vi "Teleop.vi"(0 "Call Context":T10) -> (6 "SubState 3":T4, 8 "SubState 4":T4, 9 "SubState 5":T9, 11 "Loop 3 Data":T5, 13 "Loop 4 Data":T3, 14 "SubState 0":T4=enum."driver control", 15 "Loop 1 Data":T7, 16 "Loop 0 Data":T8, 17 "SubState 1":T4, 18 "Loop 2 Data":T6, 19 "SubState 2":T4)   [LabVIEW 2013]
uses:
  typedefs/subStates.ctl
  <vilib>/Rock Robotics/WPI/DriverStation/WPI_DriverStationDerivedRobotMode.ctl
  typedefs/singleUseSubstate.ctl
  typedefs/Loop Datatypes/Loop 0 Datatype.ctl
  typedefs/Loop Datatypes/Loop 1 Datatype.ctl
  typedefs/Loop Datatypes/Loop 2 Datatype.ctl
  typedefs/Loop Datatypes/Loop 3 Datatype.ctl
  typedefs/Loop Datatypes/Loop 4 Datatype.ctl
  <vilib>/Rock Robotics/WPI/Joystick/WPI_JoystickDevRef.ctl
  <vilib>/Rock Robotics/WPI/Joystick/WPI_JoystickDeviceEnum.ctl
  typedefs/fg_typedef.ctl
  typedefs/vision enable.ctl
  <vilib>/Rock Robotics/WPI/Joystick/WPI_JoystickGetSetRefNum.vi
panel:
  out "JS3":T1
  out "Drive to DC":bool
  out "JS1":T1
  out "JS2":T1
  out "Exit Value":i32=-1
  # "Loop Data and Substates"
  # "Drive Loop"
  # "Shooter Pneumatics Loop"
  # "Pickup/Passing Belts Loop"
  # "Pickup Arm Loop"
  # "Shifter Loop"
  # "Latch Loop"
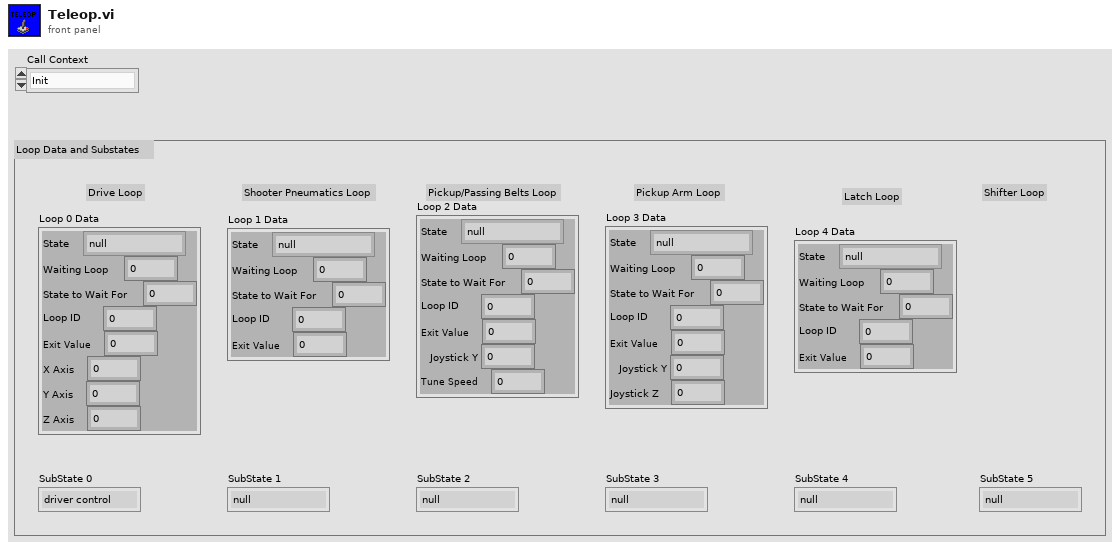
[diagram p1: front panel]
types:
  T1 = typedef "WPI_JoystickDevRef.ctl" = cluster{"Device":T2}
  T2 = typedef "WPI_JoystickDeviceEnum.ctl" = enum16{"USB 1", "USB 2", "USB 3", "USB 4", "Kinect 1", "Kinect 2"}
  T3 = typedef "Loop 4 Datatype.ctl" = cluster{"State":T4, "Waiting Loop":i32, "State to Wait For":i32, "Loop ID":i32, "Exit Value":i32}
  T4 = typedef "subStates.ctl" = enum16{"null", "wait", "driver control", "auto", "manual override", "hold position", "rotate", "pickup", "pass", "load", "goto shoot", "shoot", "end"}
  T5 = typedef "Loop 3 Datatype.ctl" = cluster{"State":T4, "Waiting Loop":i32, "State to Wait For":i32, "Loop ID":i32, "Exit Value":i32, "Joystick Y":dbl, "Joystick Z":dbl}
  T6 = typedef "Loop 2 Datatype.ctl" = cluster{"State":T4, "Waiting Loop":i32, "State to Wait For":i32, "Loop ID":i32, "Exit Value":i32, "Joystick Y":dbl, "Tune Speed":dbl}
  T7 = typedef "Loop 1 Datatype.ctl" = cluster{"State":T4, "Waiting Loop":i32, "State to Wait For":i32, "Loop ID":i32, "Exit Value":i32}
  T8 = typedef "Loop 0 Datatype.ctl" = cluster{"State":T4, "Waiting Loop":i32, "State to Wait For":i32, "Loop ID":i32, "Exit Value":i32, "X Axis":dbl, "Y Axis":dbl, "Z Axis":dbl}
  T9 = typedef "singleUseSubstate.ctl" = enum16{"null", "wait", "shift high", "shift low"}
  T10 = typedef "WPI_DriverStationDerivedRobotMode.ctl" = enum16{"Init", "Execute", "Stop"}
  T11 = cluster{"axis 1 (x)":dbl, "axis 2 (y)":dbl, "axis 3 (throttle)":dbl, "axis 4":dbl, "axis 5":dbl, "axis 6":dbl}
  T12 = typedef "WPI_EncoderDevRef.ctl" = cluster{"DevStatus":errorcluster, "EncoderIndex":T13, "CounterIndex":T14, "DistancePerCount":dbl, "Decoding Type":T15}
  T13 = typedef "FPGA_EncoderIdx.ctl" = enum8{"Enc 0", "Enc 1", "Enc 2", "Enc 3", "Invalid"}
  T14 = typedef "FPGA_CounterCtrSystemIndex.ctl" = enum8{"Ctr 0", "Ctr 1", "Ctr 2", "Ctr 3", "Ctr 4", "Ctr 5", "Ctr 6", "Ctr 7", "Invalid"}
  T15 = typedef "WPI_EncoderType.ctl" = enum16{"1x", "2x", "4x"}
  T16 = typedef "vision enable.ctl" = enum16{"Enable", "Disable", "Stop"}
  T17 = typedef "fg_typedef.ctl" = enum16{"Get", "Set"}
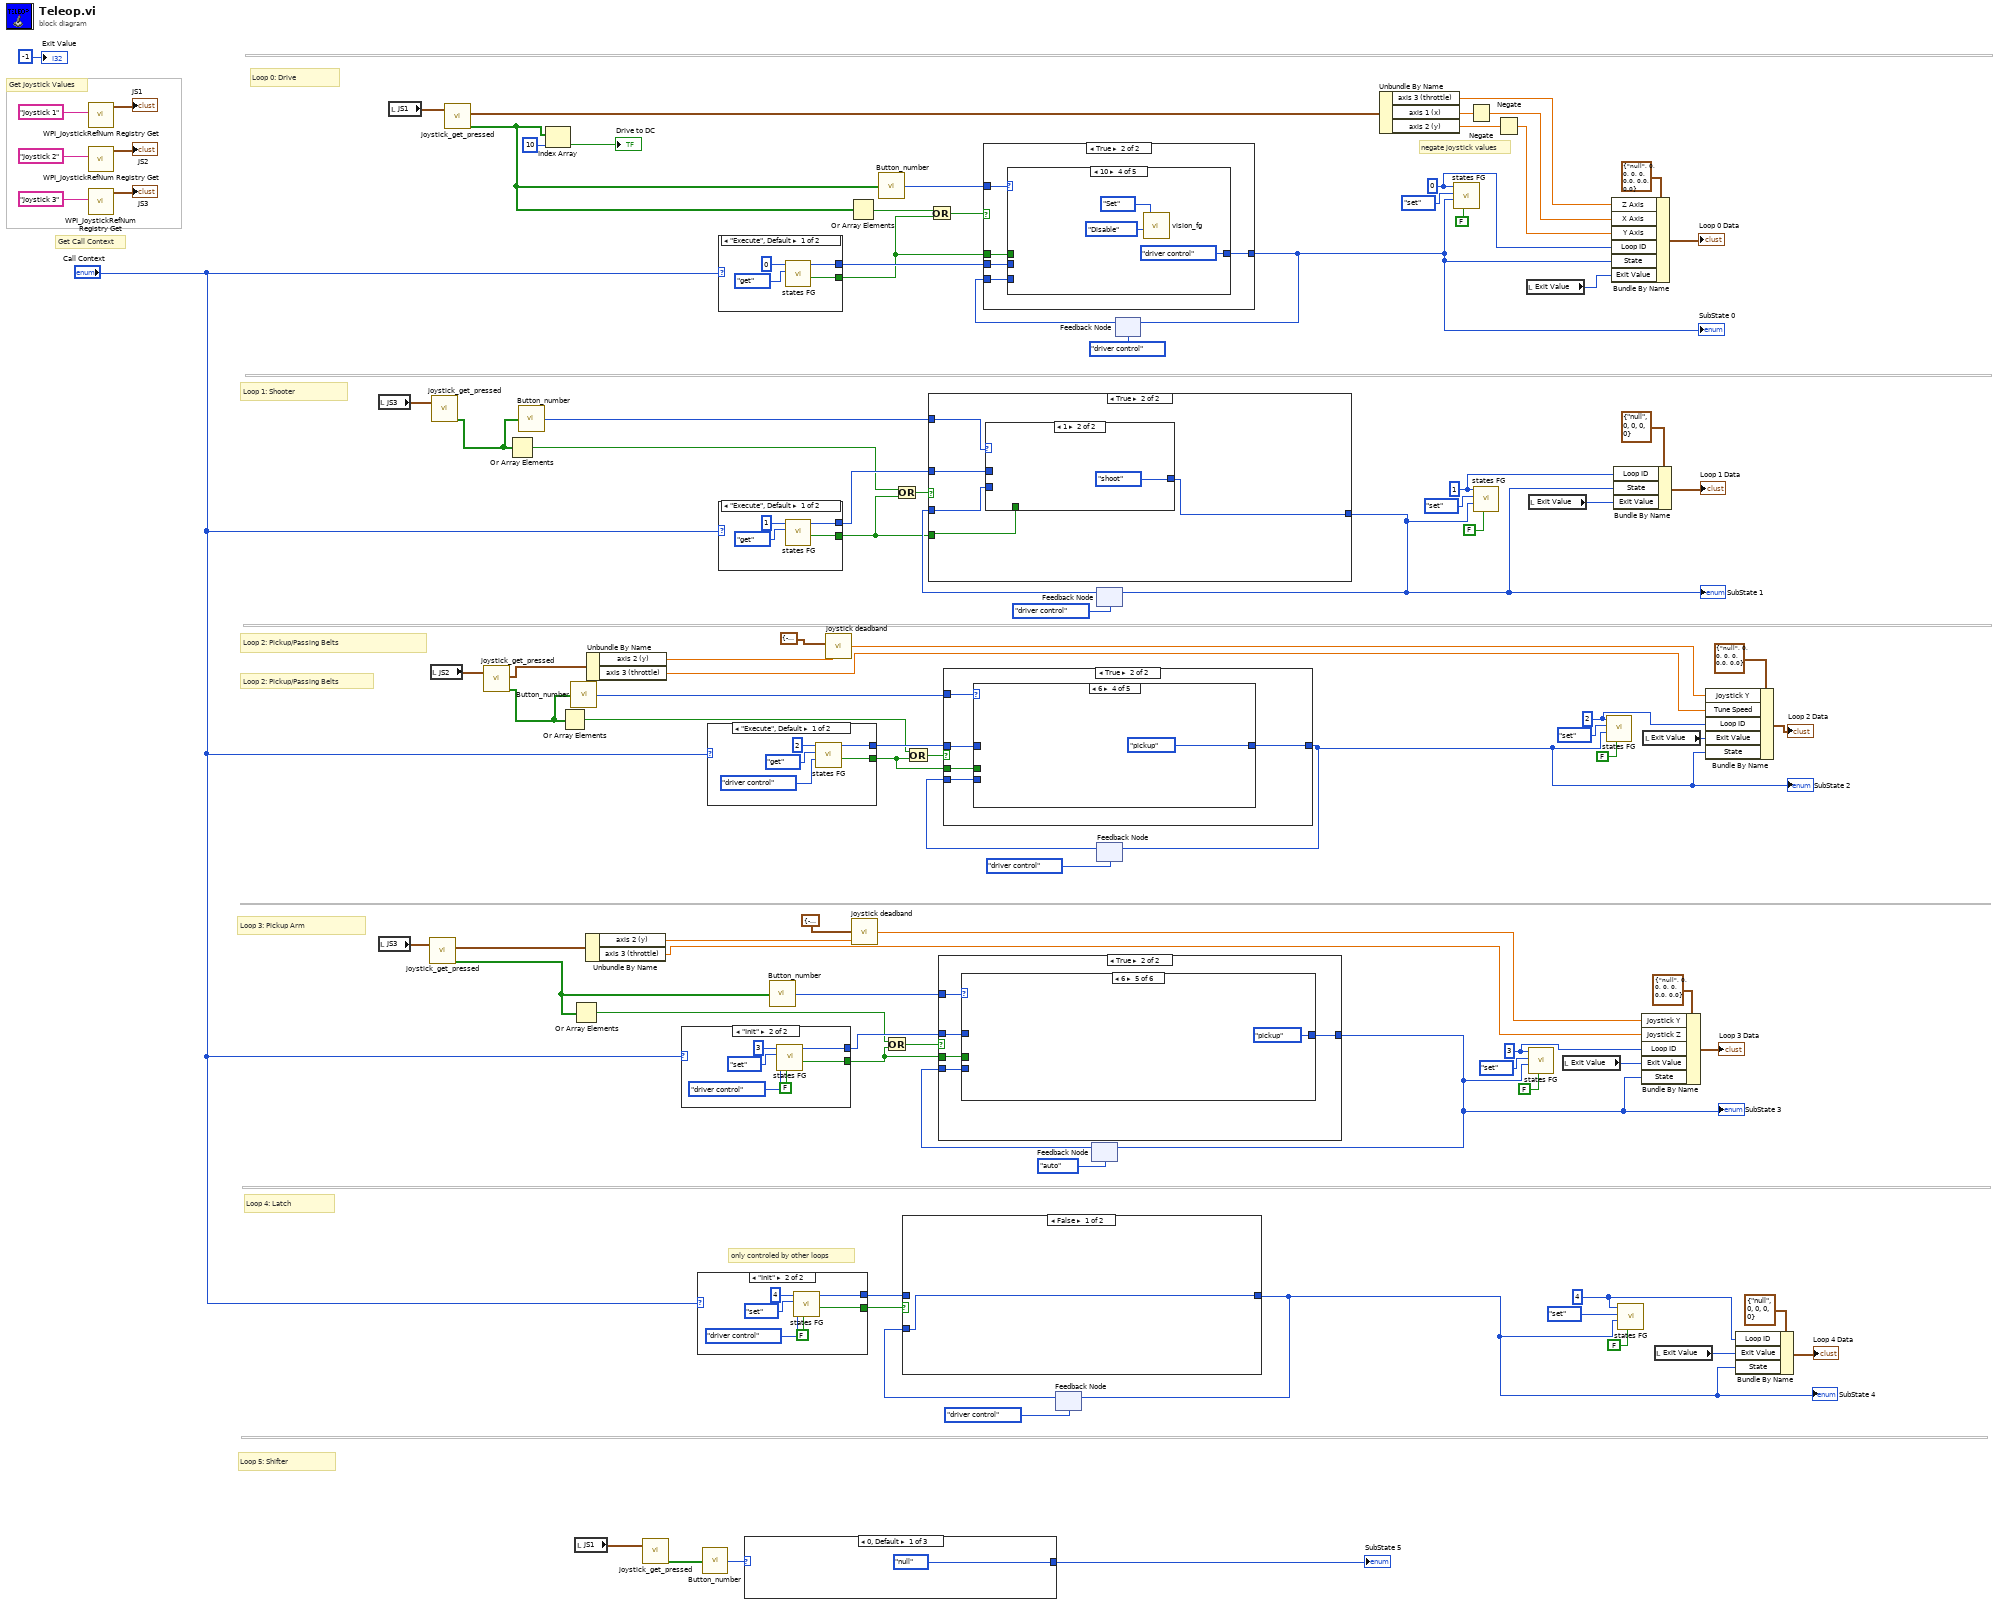
[diagram p0: block diagram]
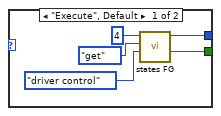
[diagram p3: hidden frame]
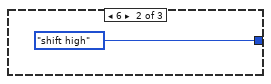
[diagram p4: hidden frame]
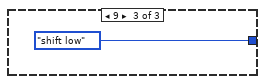
[diagram p5: hidden frame]
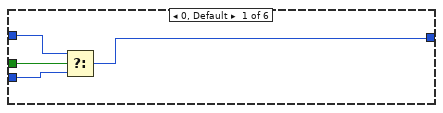
[diagram p7: hidden frame]
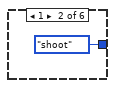
[diagram p8: hidden frame]
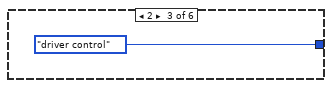
[diagram p9: hidden frame]
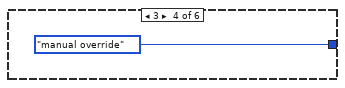
[diagram p10: hidden frame]
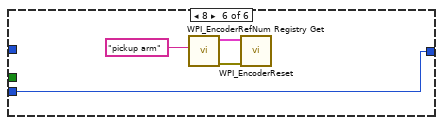
[diagram p11: hidden frame]
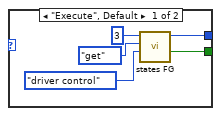
[diagram p12: hidden frame]
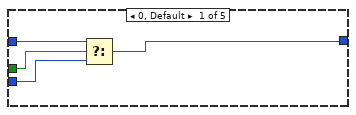
[diagram p14: hidden frame]
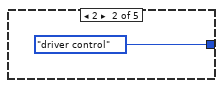
[diagram p15: hidden frame]
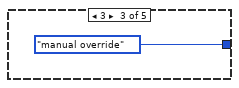
[diagram p16: hidden frame]
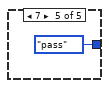
[diagram p17: hidden frame]
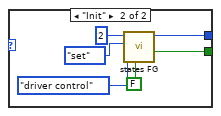
[diagram p18: hidden frame]
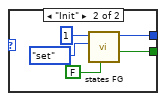
[diagram p19: hidden frame]
diagram:
  w9 = 4 ("Loop ID")
  w77 = 3 ("Loop ID")
  w78 = 2 ("Loop ID")
  w87 = 1 ("Loop ID")
  w89 = 0 ("Loop ID")
  # "only controled by other loops"
  # "Loop 2: Pickup/Passing Belts"
  # "negate joystick values"
  # "Get Call Context"
  # "Get Joystick Values"
  # "Loop 4: Latch"
  # "Loop 3: Pickup Arm"
  # "Loop 5: Shifter"
  # "Loop 2: Pickup/Passing Belts"
  # "Loop 1: Shooter"
  # "Loop 0: Drive"
  n1 = call <vilib>:"WPI_JoystickRefNum Registry Get.vi"("refnum name"="Joystick 1") -> ("JoystickDevRef"=→"JS1":T1)  [unwired: 9 in, 1 out]
  n2 = call <vilib>:"WPI_JoystickRefNum Registry Get.vi"("refnum name"="Joystick 2") -> ("JoystickDevRef"=→"JS2":T1)  [unwired: 9 in, 1 out]
  n3 = call <vilib>:"WPI_JoystickRefNum Registry Get.vi"("refnum name"="Joystick 3") -> ("JoystickDevRef"=→"JS3":T1)  [unwired: 9 in, 1 out]
  n4 = local read "JS3"() -> (w53:T1)
  n5 = local read "JS3"() -> (w38:T1)
  n6 = local read "JS1"() -> (w54:T1)
  n7 = call "joystick_get_pressed.vi"("JoystickDevRef 2"=w38) -> ("Axes"=w42:T11, "Buttons Pressed?"=w18:bool[])  [unwired: 1 in, 2 out]
  n8 = local read "JS2"() -> (w25:T1)
  n9 = call "joystick_get_pressed.vi"("JoystickDevRef 2"=w53) -> ("Buttons Pressed?"=w20:bool[])  [unwired: 1 in, 3 out]
  n10 = call "joystick_get_pressed.vi"("JoystickDevRef 2"=w54) -> ("Axes"=w58:T11, "Buttons Pressed?"=w33:bool[])  [unwired: 1 in, 2 out]
  n11 = call "joystick_get_pressed.vi"("JoystickDevRef 2"=w25) -> ("Axes"=w5:T11, "Buttons Pressed?"=w6:bool[])  [unwired: 1 in, 2 out]
  n12 = Or Array Elements(Boolean array=w20) -> (logical OR=w45:bool)
  n13 = call "Button_number.vi"("Button Array"=w20) -> ("Button Pressed"=w47:i32)
  n14 = Index Array(array=w33, index=10) -> (element=→"Drive to DC":bool)
  n15 = Or Array Elements(Boolean array=w6) -> (logical OR=w24:bool)
  n16 = call "Button_number.vi"("Button Array"=w6) -> ("Button Pressed"=w23:i32)
  n17 = Or Array Elements(Boolean array=w18) -> (logical OR=w41:bool)
  n18 = local read "JS1"() -> (w28:T1)
  n19 = Unbundle By Name(w42) -> ("axis 2 (y)"=w36:dbl, "axis 3 (throttle)"=w1:dbl)
  n20 = Unbundle By Name(w5) -> ("axis 2 (y)"=w17:dbl, "axis 3 (throttle)"=w3:dbl)
  n21 = call "joystick_get_pressed.vi"("JoystickDevRef 2"=w28) -> ("Buttons Pressed?"=w30:bool[])  [unwired: 1 in, 3 out]
  n22 = case shown="\"Init\"" "Call Context" {
    tunnel: [w108 w114] -> w39
    tunnel: [w106 w111] -> w75
    frame "Execute", Default {
      n23 = call "states FG.vi"("subState in"=subStates."driver control", "menu (get)"=enum16{"set", "get"}."get", "Loop ID"=3) -> ("exit out"=w108:bool, "subState out"=w106:T4)  [unwired: 5 in, 2 out]
    }
    frame "Init" {
      n24 = call "states FG.vi"("exit in"=FALSE, "subState in"=subStates."driver control", "menu (get)"=enum16{"set", "get"}."set", "Loop ID"=3) -> ("exit out"=w114:bool, "subState out"=w111:T4)  [unwired: 4 in, 2 out]
    }
  }
  n25 = case shown="\"Init\"" "Call Context" {
    tunnel: [w119 w125] -> w7
    tunnel: [w117 w122] -> w11
    frame "Execute", Default {
      n26 = call "states FG.vi"("subState in"=subStates."driver control", "menu (get)"=enum16{"set", "get"}."get", "Loop ID"=4) -> ("exit out"=w119:bool, "subState out"=w117:T4)  [unwired: 5 in, 2 out]
    }
    frame "Init" {
      n27 = call "states FG.vi"("exit in"=FALSE, "subState in"=subStates."driver control", "menu (get)"=enum16{"set", "get"}."set", "Loop ID"=4) -> ("exit out"=w125:bool, "subState out"=w122:T4)  [unwired: 4 in, 2 out]
    }
  }
  n28 = call "Button_number.vi"("Button Array"=w30) -> ("Button Pressed"=w29:i32)
  n29 = case shown="\"Execute\", Default" "Call Context" {
    tunnel: [w130 w136] -> w44
    tunnel: [w128 w133] -> w94
    frame "Execute", Default {
      n30 = call "states FG.vi"("subState in"=subStates."driver control", "menu (get)"=enum16{"set", "get"}."get", "Loop ID"=2) -> ("exit out"=w130:bool, "subState out"=w128:T4)  [unwired: 5 in, 2 out]
    }
    frame "Init" {
      n31 = call "states FG.vi"("exit in"=FALSE, "subState in"=subStates."driver control", "menu (get)"=enum16{"set", "get"}."set", "Loop ID"=2) -> ("exit out"=w136:bool, "subState out"=w133:T4)  [unwired: 4 in, 2 out]
    }
  }
  n32 = case shown="\"Execute\", Default" "Call Context" {
    tunnel: [w140 w145] -> w51
    tunnel: [w139 w143] -> w92
    frame "Execute", Default {
      n33 = call "states FG.vi"("menu (get)"=enum16{"set", "get"}."get", "Loop ID"=0) -> ("exit out"=w140:bool, "subState out"=w139:T4)  [unwired: 6 in, 2 out]
    }
    frame "Init" {
      n34 = call "states FG.vi"("exit in"=FALSE, "menu (get)"=enum16{"set", "get"}."set", "Loop ID"=0) -> ("exit out"=w145:bool, "subState out"=w143:T4)  [unwired: 5 in, 2 out]
    }
  }
  n35 = case shown="\"Execute\", Default" "Call Context" {
    tunnel: [w149 w154] -> w48
    tunnel: [w148 w152] -> w91
    frame "Execute", Default {
      n36 = call "states FG.vi"("menu (get)"=enum16{"set", "get"}."get", "Loop ID"=1) -> ("exit out"=w149:bool, "subState out"=w148:T4)  [unwired: 6 in, 2 out]
    }
    frame "Init" {
      n37 = call "states FG.vi"("exit in"=FALSE, "menu (get)"=enum16{"set", "get"}."set", "Loop ID"=1) -> ("exit out"=w154:bool, "subState out"=w152:T4)  [unwired: 5 in, 2 out]
    }
  }
  n38 = case shown="0, Default" w29 {
    tunnel: [singleUseSubstate."null" ("Enum") singleUseSubstate."shift high" ("Enum") singleUseSubstate."shift low" ("Enum")] -> w67
    frame 0, Default {
    }
    frame 6 {
    }
    frame 9 {
    }
  }
  "SubState 5" <- w67
  n39 = call "Button_number.vi"("Button Array"=w18) -> ("Button Pressed"=w40:i32)
  n40 = call "joystick deadband.vi"("Joystick In"=w17, "Deadband Range"=cluster{"Deadband Min":dbl, "Deadband Max":dbl} {"Deadband Min"=-0.05, "Deadband Max"=0.05}) -> ("Joystick Out"=w4:dbl)  [unwired: 4 in]
  n41 = Or Array Elements(Boolean array=w33) -> (logical OR=w52:bool)
  n42 = call "joystick deadband.vi"("Joystick In"=w36, "Deadband Range"=cluster{"Deadband Min":dbl, "Deadband Max":dbl} {"Deadband Min"=-0.05, "Deadband Max"=0.05}) -> ("Joystick Out"=w2:dbl)  [unwired: 4 in]
  n43 = call "Button_number.vi"("Button Array"=w33) -> ("Button Pressed"=w57:i32)
  n44 = Or(x=w41, y=w39) -> (x .or. y?=w43:bool)
  n45 = Or(x=w45, y=w48) -> (x .or. y?=w49:bool)
  n46 = Or(x=w24, y=w44) -> (x .or. y?=w46:bool)
  n47 = Or(x=w52, y=w51) -> (x .or. y?=w50:bool)
  n48 = feedback #1(subStates."driver control" ("Drive SubState")) -> (w14:T4)
  n49 = case shown="False" w7 {
    tunnel: w14 -> [w160 _]
    tunnel: [w160 w161] -> w37
    tunnel: w11 -> [_ w161]
    frame False {
    }
    frame True {
    }
  }
  "SubState 4" <- w37
  n50 = feedback-in #1(w37) -> ()
  n51 = feedback #2(subStates."auto" ("Drive SubState")) -> (w72:T4)
  n52 = case shown="True" w43 {
    tunnel: w72 -> [w162 w163]
    tunnel: [w162 w164] -> w59
    tunnel: w75 -> [_ w165]
    tunnel: w40 -> [_ w167]
    tunnel: w39 -> [_ w166]
    frame False {
    }
    frame True {
      n53 = case shown="6" w167 {
        tunnel: w166 -> [w171 _ _ _ _ _]
        tunnel: w163 -> [w170 _ _ _ _ w179]
        tunnel: w165 -> [w169 _ _ _ _ _]
        tunnel: [w168 subStates."shoot" ("Drive SubState") subStates."driver control" ("Drive SubState") subStates."manual override" ("Drive SubState") subStates."pickup" ("Drive SubState") w179] -> w164
        frame 0, Default {
          n54 = Select(t=w169, s=w171, f=w170) -> (s? t:f=w168:T4)
        }
        frame 1 {
        }
        frame 2 {
        }
        frame 3 {
        }
        frame 6 {
        }
        frame 8 {
          n55 = call <vilib>:"WPI_EncoderRefNum Registry Get.vi"("refnum name"="pickup arm") -> ("error out"=w177:errorcluster, "EncoderDevRef"=w176:T12)  [unwired: 9 in]
          n56 = call <vilib>:"WPI_EncoderReset.vi"("error in (no error)"=w177, "EncoderDevRef"=w176) -> ()  [unwired: 8 in, 2 out]
        }
      }
    }
  }
  "SubState 3" <- w59
  n57 = feedback-in #2(w59) -> ()
  n58 = feedback #3(subStates."driver control" ("Drive SubState")) -> (w93:T4)
  n59 = case shown="True" w49 {
    tunnel: w93 -> [w180 w184]
    tunnel: [w180 w181] -> w60
    tunnel: w91 -> [_ w185]
    tunnel: w47 -> [_ w183]
    tunnel: w48 -> [_ w182]
    frame False {
      # "nothing pressed here, move along"
    }
    frame True {
      n60 = case shown="1" w183 {
        tunnel: w185 -> [w188 _]
        tunnel: w184 -> [w187 _]
        tunnel: [w186 subStates."shoot" ("Drive SubState")] -> w181
        tunnel: w182 -> [w189 _]
        frame 0, Default {
          n61 = Select(t=w188, s=w189, f=w187) -> (s? t:f=w186:T4)
        }
        frame 1 {
        }
      }
    }
  }
  "SubState 1" <- w60
  n62 = feedback-in #3(w60) -> ()
  n63 = feedback #4(subStates."driver control" ("Drive SubState")) -> (w97:T4)
  n64 = case shown="True" w46 {
    tunnel: w97 -> [w191 w193]
    tunnel: [w191 w192] -> w16
    tunnel: w94 -> [_ w194]
    tunnel: w23 -> [_ w196]
    tunnel: w44 -> [_ w195]
    frame False {
    }
    frame True {
      n65 = case shown="6" w196 {
        tunnel: w195 -> [w200 _ _ _ _]
        tunnel: w194 -> [w199 _ _ _ _]
        tunnel: w193 -> [w198 _ _ _ _]
        tunnel: [w197 subStates."driver control" ("Drive SubState") subStates."manual override" ("Drive SubState") subStates."pickup" ("Drive SubState") subStates."pass" ("Drive SubState")] -> w192
        frame 0, Default {
          n66 = Select(t=w199, s=w200, f=w198) -> (s? t:f=w197:T4)
        }
        frame 2 {
        }
        frame 3 {
        }
        frame 6 {
        }
        frame 7 {
        }
      }
    }
  }
  "SubState 2" <- w16
  n67 = feedback-in #4(w16) -> ()
  n68 = feedback #5(subStates."driver control" ("Drive SubState")) -> (w99:T4)
  n69 = case shown="True" w50 {
    tunnel: w99 -> [w205 w207]
    tunnel: [w205 w206] -> w27
    tunnel: w92 -> [_ w208]
    tunnel: w57 -> [_ w210]
    tunnel: w51 -> [_ w209]
    frame False {
      # "keep current state, no change necessary"
    }
    frame True {
      n70 = case shown="10" w210 {
        tunnel: w209 -> [w214 _ _ _ _]
        tunnel: w208 -> [w213 _ _ _ _]
        tunnel: w207 -> [w212 w219 _ _ _]
        tunnel: [w211 w215 subStates."goto shoot" ("Drive SubState") subStates."driver control" ("Drive SubState") subStates."driver control" ("Drive SubState")] -> w206
        frame 0, Default {
          n71 = Select(t=w213, s=w214, f=w212) -> (s? t:f=w211:T4)
        }
        frame 7 {
          w216 = subStates."hold position" ("x")
          # "button 7, hold position toggle"
          n72 = Equal?(x=w216, y=w219) -> (x = y?=w218:bool)
          n73 = Select(t=subStates."driver control" ("Drive SubState"), s=w218, f=w216) -> (s? t:f=w215:T4)
        }
        frame 8 {
          # "go to shoot location"
          n74 = call "vision_fg.vi"("Action"=vision_enable."Enable", "Menu"=fg_typedef."Set") -> ()  [unwired: 1 in, 2 out]
        }
        frame 10 {
          n75 = call "vision_fg.vi"("Action"=vision_enable."Disable", "Menu"=fg_typedef."Set") -> ()  [unwired: 1 in, 2 out]
        }
        frame 11 {
          # "put robot drive in driver control"
        }
      }
    }
  }
  "SubState 0" <- w27
  n76 = feedback-in #5(w27) -> ()
  n77 = Unbundle By Name(w58) -> ("axis 3 (throttle)"=w34:dbl, "axis 1 (x)"=w64:dbl, "axis 2 (y)"=w63:dbl)
  n78 = call "states FG.vi"("exit in"=FALSE, "subState in"=w27, "menu (get)"=enum16{"set", "get"}."set", "Loop ID"=w89) -> ()  [unwired: 4 in, 4 out]
  n79 = Negate(x=w64) -> (-x=w62:dbl)
  n80 = call "states FG.vi"("exit in"=FALSE, "subState in"=w60, "menu (get)"=enum16{"set", "get"}."set", "Loop ID"=w87) -> ()  [unwired: 4 in, 4 out]
  n81 = Negate(x=w63) -> (-x=w61:dbl)
  n82 = local read "Exit Value"() -> (w85:i32)
  n83 = local read "Exit Value"() -> (w84:i32)
  n84 = call "states FG.vi"("exit in"=FALSE, "subState in"=w59, "menu (get)"=enum16{"set", "get"}."set", "Loop ID"=w77) -> ()  [unwired: 4 in, 4 out]
  n85 = local read "Exit Value"() -> (w76:i32)
  n86 = call "states FG.vi"("exit in"=FALSE, "subState in"=w16, "menu (get)"=enum16{"set", "get"}."set", "Loop ID"=w78) -> ()  [unwired: 4 in, 4 out]
  n87 = Bundle By Name(cluster=T8 {"State"=enum."null", "Waiting Loop"=0, "State to Wait For"=0, "Loop ID"=0, "Exit Value"=0, "X Axis"=0.0, "Y Axis"=0.0, "Z Axis"=0.0} ("Cluster"), "Z Axis"=w34, "X Axis"=w62, "Y Axis"=w61, "Loop ID"=w89, "State"=w27, "Exit Value"=w85) -> (→"Loop 0 Data":T8)
  n88 = Bundle By Name(cluster=T7 {"State"=enum."null", "Waiting Loop"=0, "State to Wait For"=0, "Loop ID"=0, "Exit Value"=0} ("Cluster"), "Loop ID"=w87, "State"=w60, "Exit Value"=w84) -> (→"Loop 1 Data":T7)
  n89 = call "states FG.vi"("exit in"=FALSE, "subState in"=w37, "menu (get)"=enum16{"set", "get"}."set", "Loop ID"=w9) -> ()  [unwired: 4 in, 4 out]
  n90 = Bundle By Name(cluster=T5 {"State"=enum."null", "Waiting Loop"=0, "State to Wait For"=0, "Loop ID"=0, "Exit Value"=0, "Joystick Y"=0.0, "Joystick Z"=0.0} ("Loop 3 Data"), "Joystick Y"=w2, "Joystick Z"=w1, "Loop ID"=w77, "Exit Value"=w76, "State"=w59) -> (→"Loop 3 Data":T5)
  n91 = local read "Exit Value"() -> (w79:i32)
  n92 = local read "Exit Value"() -> (w10:i32)
  n93 = Bundle By Name(cluster=T6 {"State"=enum."null", "Waiting Loop"=0, "State to Wait For"=0, "Loop ID"=0, "Exit Value"=0, "Joystick Y"=0.0, "Tune Speed"=0.0} ("Loop 2 Data"), "Joystick Y"=w4, "Tune Speed"=w3, "Loop ID"=w78, "Exit Value"=w79, "State"=w16) -> (→"Loop 2 Data":T6)
  n94 = Bundle By Name(cluster=T3 {"State"=enum."null", "Waiting Loop"=0, "State to Wait For"=0, "Loop ID"=0, "Exit Value"=0} ("Loop 4 Data"), "Loop ID"=w9, "Exit Value"=w10, "State"=w37) -> (→"Loop 4 Data":T3)
  "Exit Value" <- -1 ("Exit Value")
